vi "Table Selection Delete.vi"(9 "Filled Up String":string, 11 "Table Ref In":refnum<vi>) -> (3 "Table Ref Out":refnum<vi>)   [LabVIEW 2024]
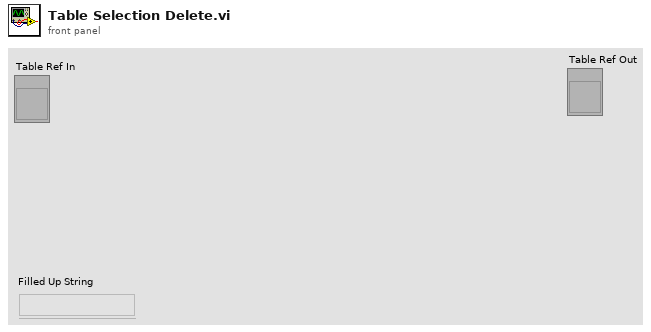
[diagram p1: front panel]
types:
  T1 = typedef "LVRowAndColumnTypeDef.ctl" = cluster{"Row":i32, "Column":i32}
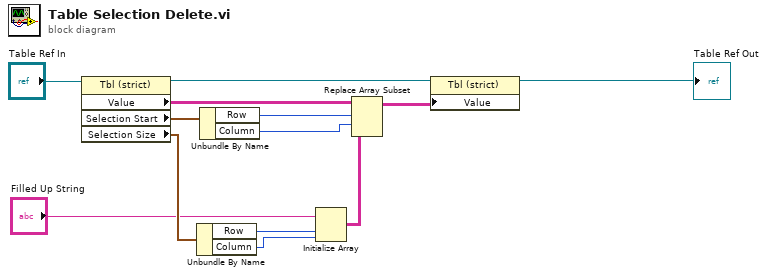
[diagram p0: block diagram]
diagram:
  n1 = property class="Tbl (strict)"(reference="Table Ref In") -> (reference out=w10:refnum<vi>, "Value"=w8:string[][], "Selection Start"=w13:T1, "Selection Size"=w12:T1)  [unwired: 1 in, 1 out]
  n2 = Unbundle By Name(w12) -> ("Row"=w4:i32, "Column"=w3:i32)
  n3 = Unbundle By Name(w13) -> ("Row"=w7:i32, "Column"=w6:i32)
  n4 = Initialize Array("Filled Up String", w4, w3) -> (w2:string[][])
  n5 = Replace Array Subset(array=w8, new element=w2, index (row)=w7, index (col)=w6) -> (w5:string[][])
  n6 = property class="Tbl (strict)"(reference=w10, "Value"=w5) -> (reference out=→"Table Ref Out":refnum<vi>)  [unwired: 1 in, 1 out]
